vi "LV to DAT 2D.vi"(4 "append to file? (new file:F)":bool, 6 "wavenames (.Vx, etc)":string[](array[string]), 7 "filename":string, 8 "error in":errorcluster, 9 "Data":dbl[][](array[numeric]), 10 "Comments":string, 11 "path":path) -> (0 "error out":errorcluster, 3 "new file path":path)   [LabVIEW 2016, in "LVtoITX.lvclass"]
uses:
  LVtoITX.lvclass
  <vilib>/Utility/file.llb/Write Delimited Spreadsheet (DBL).vi
  <vilib>/Utility/file.llb/Write Delimited Spreadsheet (string).vi
panel:
  out "appended array":string[][](array[string])
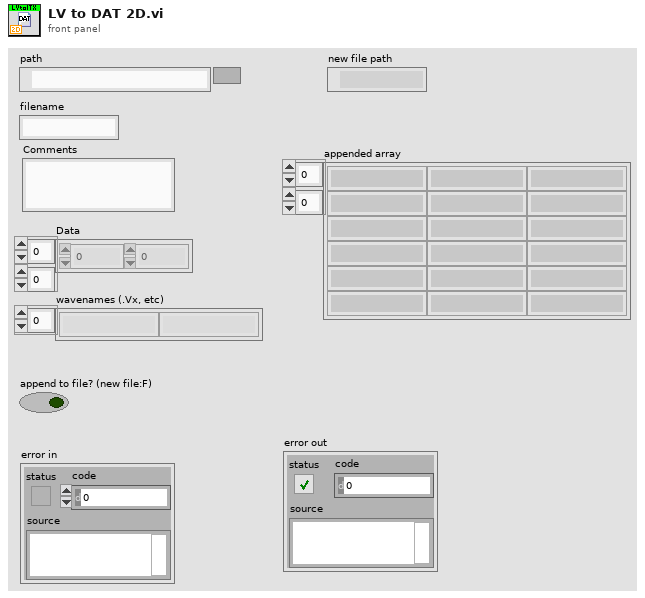
[diagram p1: front panel]
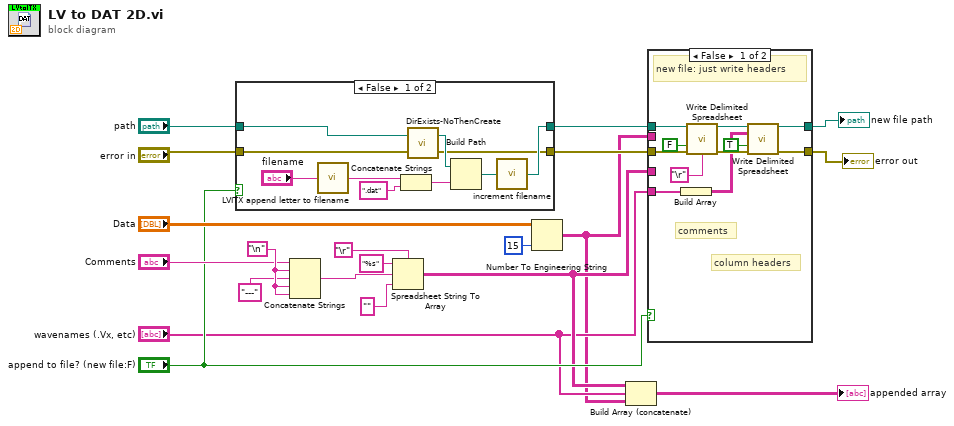
[diagram p0: block diagram]
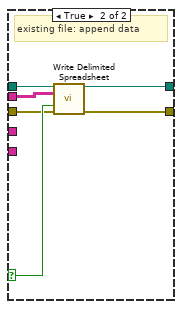
[diagram p2: hidden frame]
diagram:
  w13 = "\n"
  n1 = case shown="False" "append to file? (new file:F)" {
    tunnel: [w30 w32] -> w9
    tunnel: "path" -> [w28 w32]
    tunnel: "error in" -> [w22 w31]
    tunnel: [w21 w31] -> w8
    frame False {
      n2 = call "LVITX append letter to filename.vi"("string in"="filename") -> ("string out"=w23:string)
      n3 = Concatenate Strings(w23, ".dat" ("string")) -> (w24:string)
      n4 = call <userlib>:"DirExists-NoThenCreate.vi"("error in"=w22, "path"=w28) -> ("error out"=w21:errorcluster, "created path"=w25:path)
      n5 = Build Path(base path=w25, name or relative path=w24) -> (appended path=w26:path)
      n6 = call <userlib>:"increment filename.vi"("path"=w26) -> ("modified path"=w30:path)
    }
    frame True {
    }
  }
  n7 = Concatenate Strings("Comments", w13, "---" ("string"), w13, w13) -> (w14:string)
  n8 = Spreadsheet String To Array(delimiter (Tab)="\r", format string="%s", spreadsheet string=w14, array type (2D Dbl)="") -> (array=w4:string[][])
  n9 = Number To Engineering String(2:i16 15 ("precision (6)"), 4:"Data") -> (0:w2:string[][])  [unwired: 2 out]
  n10 = Build Array (concatenate)(w4, "wavenames (.Vx, etc)", w2) -> (→"appended array":string[][])
  n11 = case shown="False" "append to file? (new file:F)" {
    selector: "append to file? (new file:F)" -> [_ w48]
    tunnel: [w41 w46] -> w6
    tunnel: w9 -> [w43 w49]
    tunnel: w8 -> [w42 w47]
    tunnel: [w38 w45] -> w7
    tunnel: w2 -> [_ w44]
    tunnel: "wavenames (.Vx, etc)" -> [w33 _]
    tunnel: w4 -> [_ _]
    frame False {
      # "column headers"
      # "comments"
      # "new file: just write headers"
      n12 = Build Array(w33) -> (w34:string[][])
      n13 = call-poly <vilib>:"Write Delimited Spreadsheet.vi"("file path (dialog if empty)"=w43, "append to file? (new file:F)"=FALSE, "error in (no error)"=w42, "delimiter (\\t)"="\r") -> ("new file path (Not A Path if cancelled)"=w39:path, "error out"=w40:errorcluster)  [unwired: 10 in]
      n14 = call-poly <vilib>:"Write Delimited Spreadsheet.vi"("file path (dialog if empty)"=w39, "2D data"=w34, "append to file? (new file:F)"=TRUE, "error in (no error)"=w40) -> ("new file path (Not A Path if cancelled)"=w41:path, "error out"=w38:errorcluster)  [unwired: 10 in]
    }
    frame True {
      # "existing file: append data"
      n15 = call-poly <vilib>:"Write Delimited Spreadsheet.vi"("file path (dialog if empty)"=w49, "2D data"=w44, "append to file? (new file:F)"=w48, "error in (no error)"=w47) -> ("new file path (Not A Path if cancelled)"=w46:path, "error out"=w45:errorcluster)  [unwired: 10 in]
    }
  }
  "new file path" <- w6
  "error out" <- w7
